vi "Rename Destination.vi"(8 "error in (no error)":errorcluster, 9 "New name":string, 10 "Old name":string, 11 "SigMan in":refnum<class "SignalManager.lvclass">) -> (0 "error out":errorcluster, 3 "SigMan out":refnum<class "SignalManager.lvclass">)   [LabVIEW 2015, in "SignalManager.lvclass"]
uses:
  SignalManager.lvclass
  SignalManager.lvclass/SignalManager.ctl
  Channel/Channel.lvclass/Channel.ctl
  Channel/Write Destination.vi
  Channel/Read Destination.vi
  Channel/Channel.lvclass
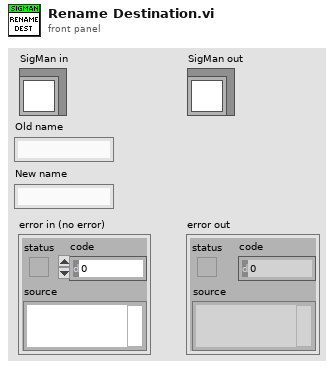
[diagram p1: front panel]
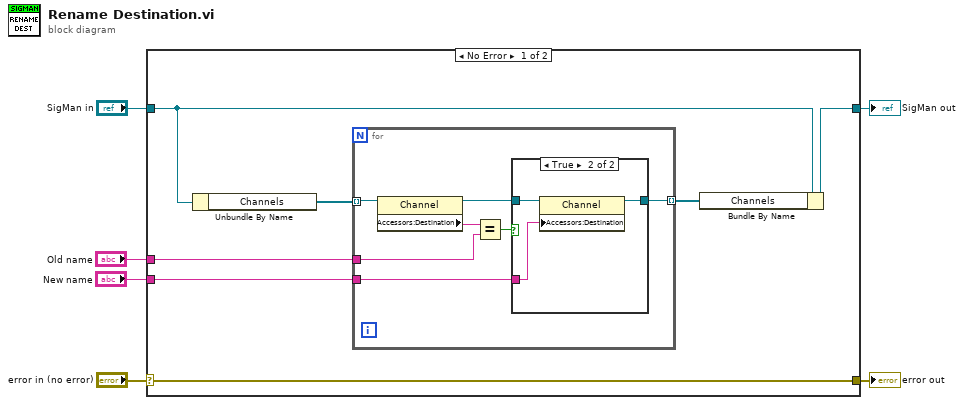
[diagram p0: block diagram]
diagram:
  n1 = case shown="No Error" "error in (no error)" {
    selector: "error in (no error)" -> [w13 w26]
    tunnel: [w13 w26] -> w5
    tunnel: [w9 w25] -> w3
    tunnel: "SigMan in" -> [w11 w25]
    tunnel: "Old name" -> [w10 _]
    tunnel: "New name" -> [w7 _]
    frame No Error {
      n2 = Unbundle By Name(w11) -> ("Channels"=w12:refnum<class "Channel.lvclass">[])
      n3 = for {
        tunnel: w12 -> [w20] mode=indexing
        tunnel: w10 -> [w17]
        tunnel: [w15] -> w8 mode=indexing
        tunnel: w7 -> [w14]
        n4 = property class="Channel"(reference=w20) -> (reference out=w16:refnum<class "Channel.lvclass">, "Accessors:Destination"=w18:string)  [unwired: 1 in, 1 out]
        n5 = Equal?(x=w18, y=w17) -> (x = y?=w19:bool)
        n6 = case shown="True" w19 {
          tunnel: w16 -> [w21 w24]
          tunnel: [w21 w23] -> w15
          tunnel: w14 -> [_ w22]
          frame False {
          }
          frame True {
            n7 = property class="Channel"(reference=w24, "Accessors:Destination"=w22) -> (reference out=w23:refnum<class "Channel.lvclass">)  [unwired: 1 in, 1 out]
          }
        }
      }
      n8 = Bundle By Name(cluster=w11, "Channels"=w8) -> (w9:refnum<class "SignalManager.lvclass">)
    }
    frame Error {
    }
  }
  "error out" <- w5
  "SigMan out" <- w3
